vi "SIM Set Node Discrete Rate.vi"(8 "error in (no error)":errorcluster, 9 "skew (0)":dbl, 10 "period (auto)":dbl=-1.0, 11 "node ref":refnum<vi>) -> (0 "error out":errorcluster, 2 "succeeded":bool, 3 "dup node ref":refnum<vi>)   [LabVIEW 2017]
panel:
  # "Auto Discrete Period will execute every time a discrete timestep is taken. This \nwill either be at the base discrete rate configured in the simulation or at a \nthe greatest common denominator of all discrete rates configured on other \nnodes in the Simulation."
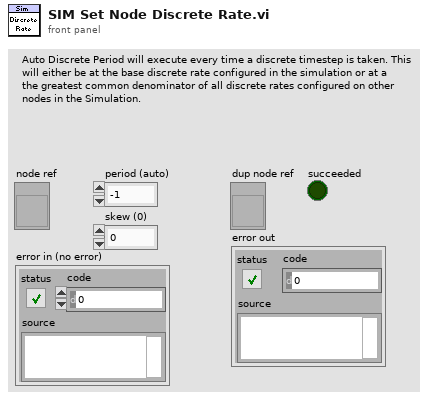
[diagram p1: front panel]
types:
  T1 = enum16{"Function call", "Discrete", "Continuous", "Initialization only", "Final step only"}
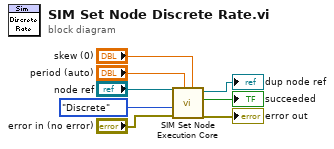
[diagram p0: block diagram]
diagram:
  n1 = call <vilib>:"SIM Set Node Execution Core.vi"("skew (0)"="skew (0)", "period (auto)"="period (auto)", "error in (no error)"="error in (no error)", "execution type (continuous)"=T1."Discrete", "Node in"="node ref") -> ("error out"=→"error out":errorcluster, "succeeded"=→"succeeded":bool, "Node out"=→"dup node ref":refnum<vi>)  [unwired: 4 in]
